vi "LoggingLoop.vi"(8 "Error In":errorcluster, 11 "Message Queues":T1) -> (0 "Error Out":errorcluster)   [LabVIEW 2017, in "Server.lvlib" / "Logging.lvlib"]
doc: "This Loop accepts \"Log\"-Messages with LogData.ctl as Datatype. It then logs the Type of Message, the Message Data and the Timestamp of the message to a tdms-file."
uses:
  Logging.lvlib
  Message Queue/CommReferences.ctl
  Message Queue/MessageCluster.ctl
  LoggingLoopData.ctl
  TypeDefs/ServerINI.ctl
  Oracle/OracleData.ctl
  LogData.ctl
  <vilib>/Utility/error.llb/Error Cluster From Error Code.vi
  <vilib>/ErrorRing/Error Ring.xnode
  Message Queue/Message Queue.lvlib
  ErrorLogger/ErrorLogger.lvlib
  Oracle/Oracle.lvlib
  Server.lvlib
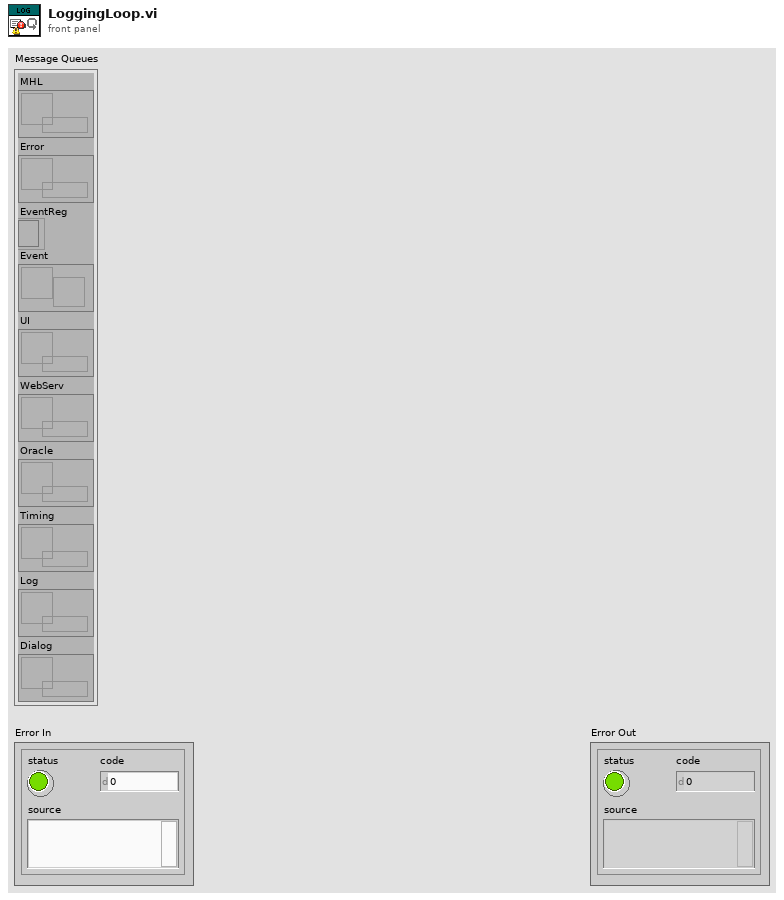
[diagram p1: front panel]
types:
  T1 = typedef "Server.lvlib/Message Queue.lvlib/CommReferences.ctl" = cluster{"MHL":refnum<queue>, "Error":refnum<queue>, "EventReg":refnum<event-registration>, "Event":refnum<user-event>, "UI":refnum<queue>, "WebServ":refnum<queue>, "Oracle":refnum<queue>, "Timing":refnum<queue>, "Log":refnum<queue>, "Dialog":refnum<queue>}
  T2 = typedef "Server.lvlib/Logging.lvlib/LoggingLoopData.ctl" = cluster{"TDMS Ref":refnum<k34>, "LogPath":path}
  T3 = typedef "Server.lvlib/ServerINI.ctl" = cluster{"ClientTimeout (s)":u32, "LogPath":path, "CriticalErrors":i32[], "OracleData":T4}
  T4 = typedef "Server.lvlib/Oracle.lvlib/OracleData.ctl" = cluster{"DBname":string, "User":string, "Password":string}
  T5 = enum16{"open", "open or create", "create or replace", "create", "open (read-only)"}
  T6 = typedef "Server.lvlib/Logging.lvlib/LogData.ctl" = cluster{"Time":timestamp, "Type":string, "LogText":string}
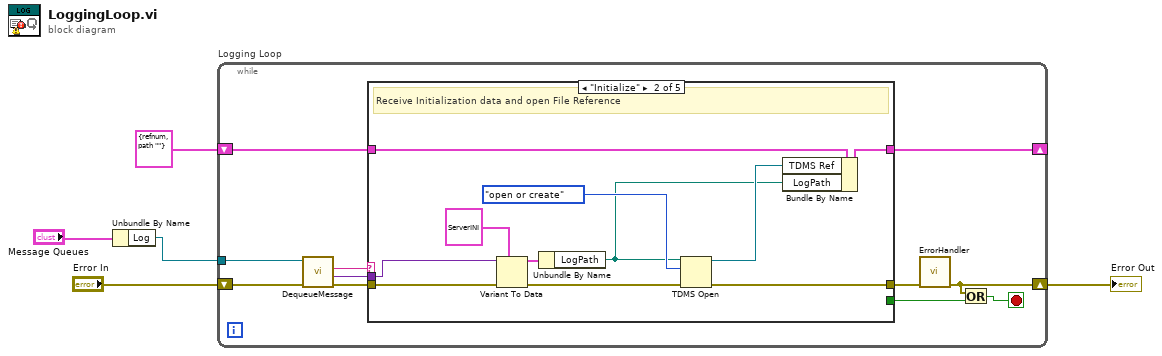
[diagram p0: block diagram]
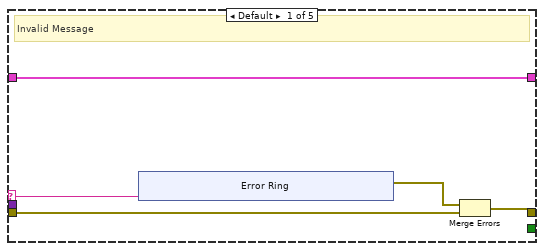
[diagram p2: hidden frame]
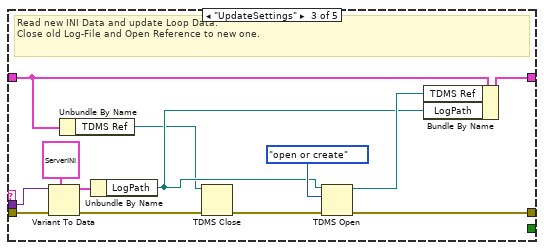
[diagram p3: hidden frame]
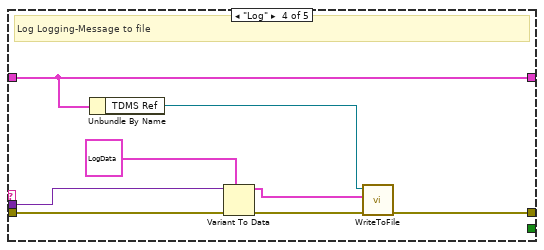
[diagram p4: hidden frame]
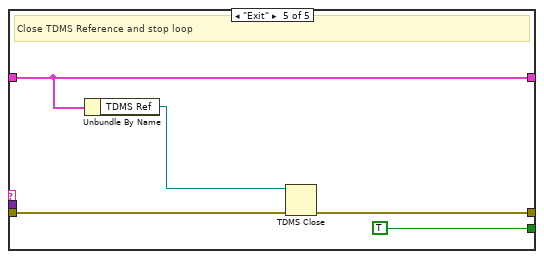
[diagram p5: hidden frame]
diagram:
  n1 = Unbundle By Name("Message Queues") -> ("Log"=w2:refnum<queue>)
  n2 = while "Logging Loop" {
    shift-right: [w6] -> w4
    shift-left: "Error In" -> [w16]
    tunnel: w2 -> [w8]
    shift-right: [w9] -> _
    shift-left: T2 {"TDMS Ref"=refnum, "LogPath"=path ""} ("LoggingLoopData") -> [w10]
    stop <- w7 stop-if-true
    n3 = call "DequeueMessage.vi"("error in (no error)"=w16, "Message Queue"=w8) -> ("error out"=w15:errorcluster, "Message Data"=w12:variant, "Message"=w13:string)  [unwired: 5 in, 2 out]
    n4 = case shown="\"Initialize\"" w13 {
      selector: w13 -> [w20 _ _ _ _]
      tunnel: [w19 w38 w51 w56 w63] -> w14
      tunnel: w15 -> [w21 w39 w52 w60 w65]
      tunnel: w12 -> [_ w34 w48 w58 _]
      tunnel: [_ _ _ _ TRUE] -> w11
      tunnel: [w17 w32 w46 w54 w62] -> w9
      tunnel: w10 -> [w17 w36 w42 w54 w62]
      frame Default {
        # "Invalid Message"
        n5 = xnode "Error Ring"("parameter 0"=w20) -> ("error out"=w18:errorcluster)
        n6 = Merge Errors(w18, w21) -> (w19:errorcluster)
      }
      frame "Initialize" {
        # "Receive Initialization data and open File Reference"
        n7 = Variant To Data(error in=w39, type=T3 {"ClientTimeout (s)"=30, "LogPath"=path "C:/Users/jgoebel/Documents/GitHub/AEDashboard/ServerLib/Data/ServerLog.tdms", "CriticalErrors"=[], "OracleData"={"DBname"="", "User"="", "Password"=""}} ("ServerINI"), Variant=w34) -> (data=w30:T3, error out=w35:errorcluster)
        n8 = Unbundle By Name(w30) -> ("LogPath"=w29:path)
        n9 = TDMS Open(8:w35, 10:T5."open or create" ("operation (0:open)"), 11:w29) -> (0:w38:errorcluster, 3:w31:refnum<k34>)  [unwired: 4 in]
        n10 = Bundle By Name(cluster=w36, "TDMS Ref"=w31, "LogPath"=w29) -> (w32:T2)
      }
      frame "UpdateSettings" {
        # "Read new INI Data and update Loop Data.\nClose old Log-File and Open Reference to new one."
        n11 = Variant To Data(error in=w52, type=T3 {"ClientTimeout (s)"=30, "LogPath"=path "C:/Users/jgoebel/Documents/GitHub/AEDashboard/ServerLib/Data/ServerLog.tdms", "CriticalErrors"=[], "OracleData"={"DBname"="", "User"="", "Password"=""}} ("ServerINI"), Variant=w48) -> (data=w44:T3, error out=w49:errorcluster)
        n12 = Unbundle By Name(w42) -> ("TDMS Ref"=w40:refnum<k34>)
        n13 = Unbundle By Name(w44) -> ("LogPath"=w43:path)
        n14 = TDMS Close(8:w49, 11:w40) -> (0:w41:errorcluster)  [unwired: 1 out]
        n15 = TDMS Open(8:w41, 10:T5."open or create" ("operation (0:open)"), 11:w43) -> (0:w51:errorcluster, 3:w45:refnum<k34>)  [unwired: 4 in]
        n16 = Bundle By Name(cluster=w42, "TDMS Ref"=w45, "LogPath"=w43) -> (w46:T2)
      }
      frame "Log" {
        # "Log Logging-Message to file"
        n17 = Unbundle By Name(w54) -> ("TDMS Ref"=w53:refnum<k34>)
        n18 = Variant To Data(error in=w60, type=T6 {"Time"=timestamp(0 s since 1904-01-01), "Type"="", "LogText"=""} ("LogData"), Variant=w58) -> (data=w55:T6, error out=w59:errorcluster)
        n19 = call "WriteToFile.vi"("error in (no error)"=w59, "LogData"=w55, "Refnum in"=w53) -> ("error out"=w56:errorcluster)  [unwired: 7 in, 1 out]
      }
      frame "Exit" {
        # "Close TDMS Reference and stop loop"
        n20 = Unbundle By Name(w62) -> ("TDMS Ref"=w61:refnum<k34>)
        n21 = TDMS Close(8:w65, 11:w61) -> (0:w63:errorcluster)  [unwired: 1 out]
      }
    }
    n22 = call "ErrorHandler.vi"("error in (no error)"=w14) -> ("error out"=w6:errorcluster)  [unwired: 10 in]
    n23 = Or(x=w6, y=w11) -> (x .or. y?=w7:bool)
  }
  "Error Out" <- w4
